vi "Do.vi"(8 "error in (no error)":errorcluster, 10 "Actor in":refnum<class "Actor.lvclass">, 11 "Conceret Initialize Create Sensor Msg in":refnum<class "Conceret Initialize Create Sensor Msg.lvclass">) -> (0 "error out":errorcluster, 2 "Actor out":refnum<class "Actor.lvclass">)   [LabVIEW 2013, in "Create Sensor View.lvlib" / "Conceret Initialize Create Sensor Msg.lvclass"]
doc: "(<B>Filename</B>: Actor Framework.lvlib:Message.lvclass:Do.vi)\n\nDefines what a message does when it is received by an actor. Generally, a message instructs an actor to invoke one of its methods.\n\nBy default, this method does nothing. A child class must override it to define behavior. Create a child class by using the Actor Framework Message Maker dialog box."
uses:
  Conceret Initialize Create Sensor Msg.lvclass
  <vilib>/ActorFramework/Actor/Actor.lvclass
  Create Sensor View/Create Sensor View.lvclass
  Models/Create Sensor Model Messages/Abstract Initialize Create Sensor Msg/Abstract Initialize Create Sensor Msg.lvclass
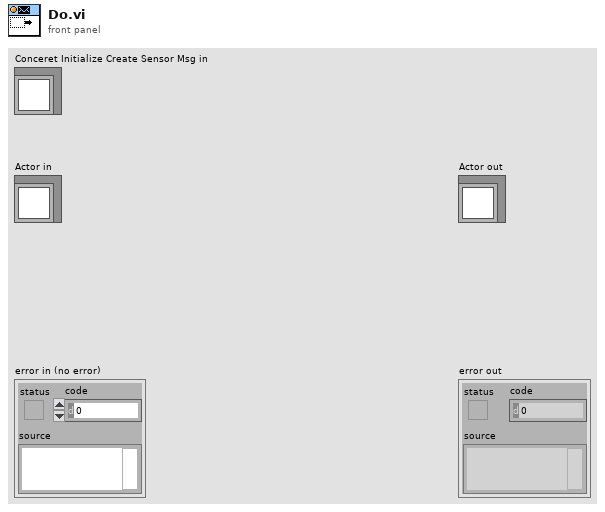
[diagram p1: front panel]
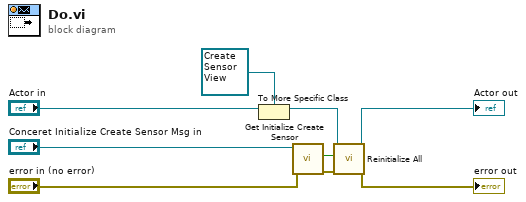
[diagram p0: block diagram]
diagram:
  n1 = To More Specific Class(target class=refnum<class "Create Sensor View.lvclass"> refnum ("Create Sensor View.lvlib:Create Sensor View.lvclass"), reference="Actor in") -> (specific class reference=w6:refnum<class "Create Sensor View.lvclass">)  [unwired: 1 in, 1 out]
  n2 = call "Get Initialize Create Sensor.vi"("error in (no error)"="error in (no error)", "Abstract Initialize Create Sensor Msg in"="Conceret Initialize Create Sensor Msg in") -> ("error out"=w5:errorcluster, "Initialize Create Sensor"=w1:bool)  [unwired: 7 in, 1 out]
  n3 = call "Reinitialize All.vi"("error in (no error)"=w5, "Initialize Create Sensor"=w1, "Create Sensor View in"=w6) -> ("error out"=→"error out":errorcluster, "Create Sensor View out"=→"Actor out":refnum<class "Create Sensor View.lvclass">)  [unwired: 7 in]
